vi "Edit Config.vi"(8 "error in (no error)":errorcluster, 11 "Multi Parser in":refnum<class "Mulit Sentence Parser.lvclass">) -> (0 "error out":errorcluster, 3 "Multi Parser out":refnum<class "Mulit Sentence Parser.lvclass">)   [LabVIEW 2018, in "Mulit Sentence Parser.lvclass"]
doc: "Multi Sentence Parser.lvclass:Edit Config.vi\n\nThis VI is used to edit the Multi Sentence Parser configuration parameters.\n\nInstrument Communication Module Version 1.0\nOctober, 2017 Original Code Consulting David Thomson\n www.originalcode.com"
uses:
  Mulit Sentence Parser.lvclass
  Multi Sentence Parser Config.ctl
  Controls/ICM Class Editor State.ctl
  Controls/ICM Editor Command.ctl
  Mulit Sentence Parser.lvclass/Mulit Sentence Parser.ctl
panel:
  in  "Save":bool
  in  "Revert":bool
  in  "Multi Sentence Parser Config":T1
  # "This Parser is intended to be used with devices which send multiple data sentences, potentially at different intervals."
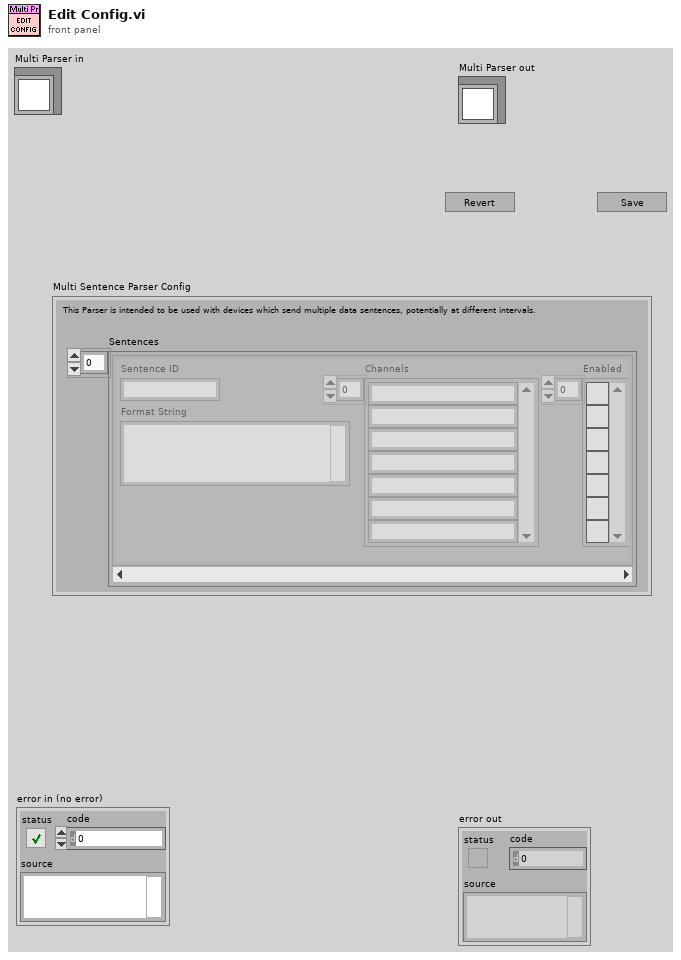
[diagram p1: front panel]
types:
  T1 = typedef "Mulit Sentence Parser.lvclass/Multi Sentence Parser Config.ctl" = cluster{"Sentences":cluster{"Sentence ID":string, "Format String":string, "Channels":string[], "Enabled":bool[]}[]}
  T2 = typedef "ICM Editor Command.ctl" = enum16{"No-op", "Exit"}
  T3 = typedef "ICM Class Editor State.ctl" = enum16{"Init", "Wait", "Write", "Read", "Display", "Set Flashing", "Error", "Stop"}
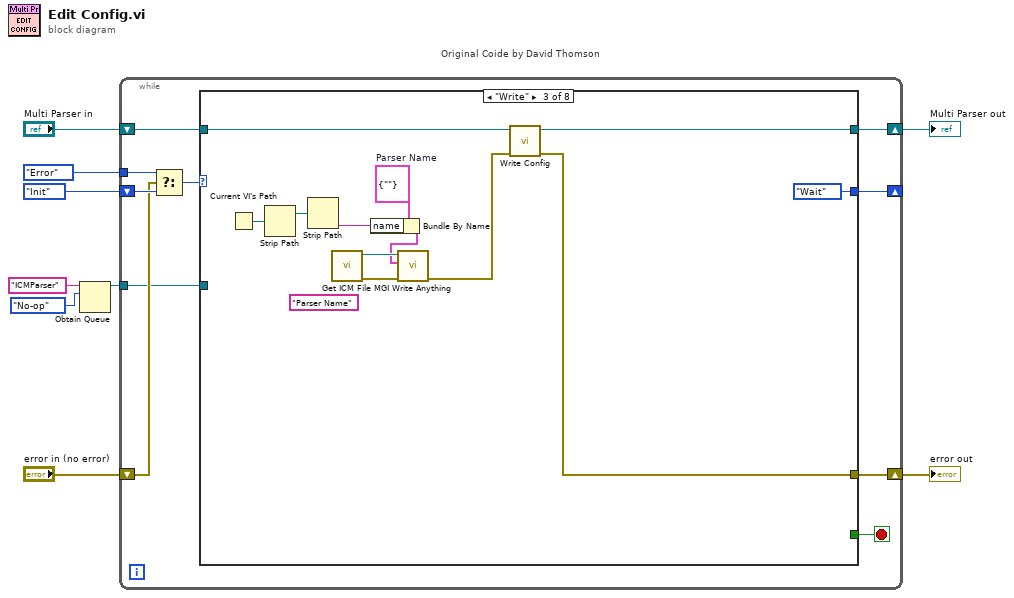
[diagram p0: block diagram]
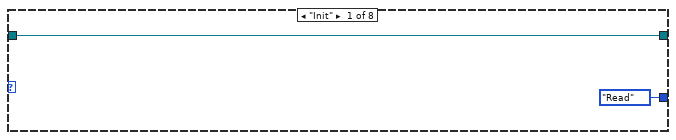
[diagram p2: hidden frame]
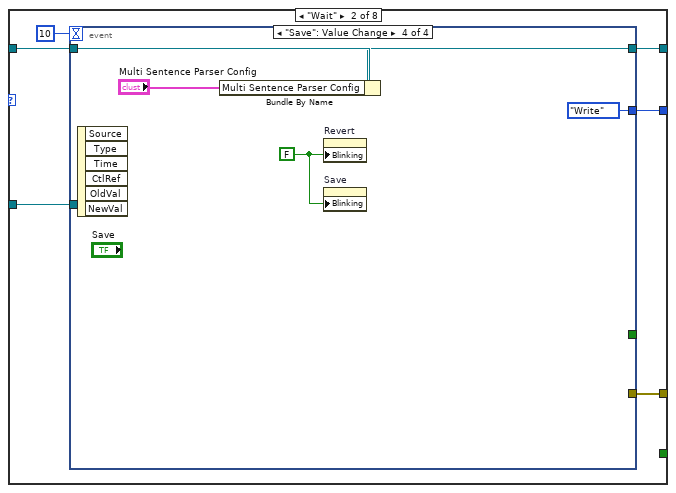
[diagram p3: hidden frame]
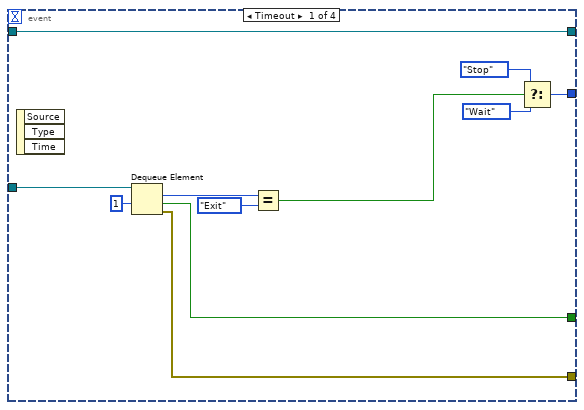
[diagram p4: hidden frame]
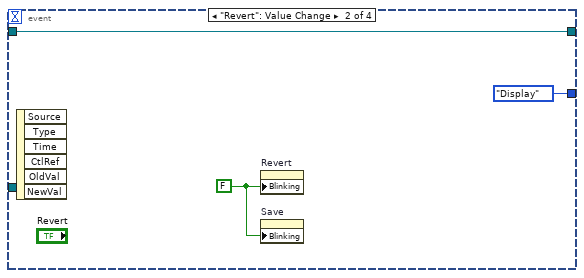
[diagram p5: hidden frame]
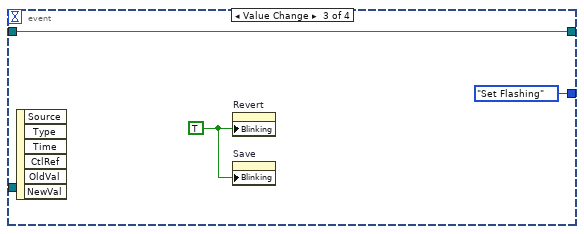
[diagram p6: hidden frame]
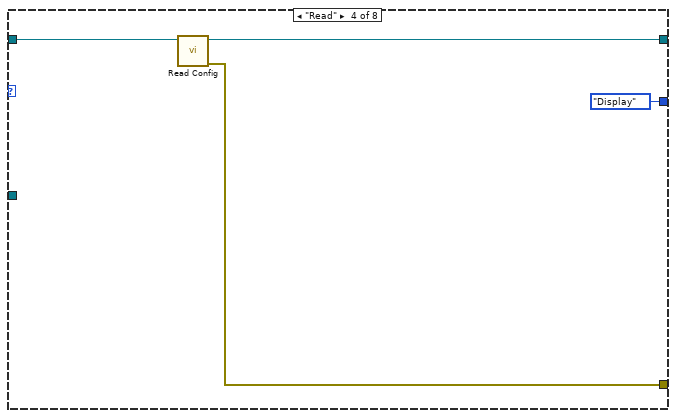
[diagram p7: hidden frame]
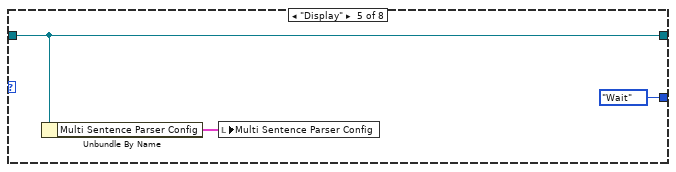
[diagram p8: hidden frame]
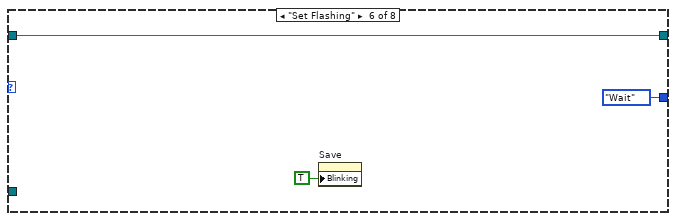
[diagram p9: hidden frame]
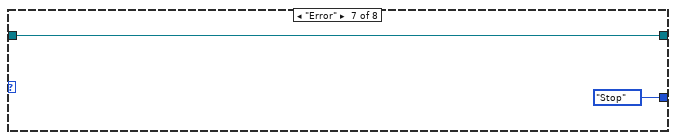
[diagram p10: hidden frame]
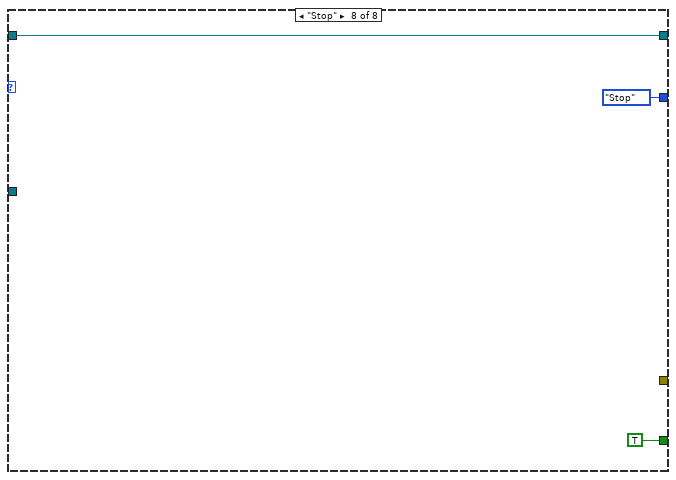
[diagram p11: hidden frame]
diagram:
  n1 = Obtain Queue(name (unnamed)="ICMParser", element data type=ICM_Editor_Command."No-op" ("Editor Command")) -> (queue out=w1:refnum<queue>)  [unwired: 3 in, 2 out]
  n2 = while "Original Coide by David Thomson" {
    shift-right: [w19] -> w8
    shift-left: "Multi Parser in" -> [w18]
    shift-right: [w12] -> _
    shift-left: ICM_Class_Editor_State."Init" ("Config State") -> [w16]
    shift-right: [w11] -> w6
    shift-left: "error in (no error)" -> [w14]
    tunnel: ICM_Class_Editor_State."Error" ("Config State") -> [w13]
    tunnel: w1 -> [w10]
    stop <- w17 stop-if-true
    n3 = Select(t=w13, s=w14, f=w16) -> (s? t:f=w15:T3)
    n4 = case shown="\"Write\"" w15 {
      tunnel: [w20 w25 w59 w63 w68 w71 w73 w76] -> w19
      tunnel: w18 -> [w20 w24 w60 w65 w68 w71 w73 w76]
      tunnel: [_ _ _ _ _ _ _ TRUE] -> w17
      tunnel: [ICM_Class_Editor_State."Read" ("Config State") w26 ICM_Class_Editor_State."Wait" ("Config State") ICM_Class_Editor_State."Display" ("Config State") ICM_Class_Editor_State."Wait" ("Config State") ICM_Class_Editor_State."Wait" ("Config State") ICM_Class_Editor_State."Stop" ("Config State") ICM_Class_Editor_State."Stop" ("Config State")] -> w12
      tunnel: [_ w22 w58 w64 _ _ _ _] -> w11
      tunnel: w10 -> [_ w23 _ _ _ _ _ _]
      frame "Init" {
      }
      frame "Wait" {
        n5 = event shown="[3] \"Save\": Value Change" {
          selector: _ -> [_ _ _ _]
          dyn-events: _ -> [_ _ _ _]
          timeout: 10 -> [_ _ _ _]
          tunnel: [w35 ICM_Class_Editor_State."Display" ("Config State") ICM_Class_Editor_State."Set Flashing" ("Config State") ICM_Class_Editor_State."Write" ("Config State")] -> w26
          tunnel: [w38 w40 w44 w46] -> w25
          tunnel: w24 -> [w38 w40 w44 w47]
          tunnel: w23 -> [w37 _ _ _]
          tunnel: [w29 _ _ _] -> w22
          tunnel: [w28 _ _ _] -> _
          event Timeout {
            n6 = event-data() -> ()  [unwired: 1 in, 3 out]
            n7 = Dequeue Element(queue=w37, timeout in ms (-1)=1) -> (element=w34:T2, timed out?=w28:bool, error out=w29:errorcluster)  [unwired: 1 in, 1 out]
            n8 = Equal?(x=w34, y=ICM_Editor_Command."Exit") -> (x = y?=w32:bool)
            n9 = Select(t=ICM_Class_Editor_State."Stop" ("Config State"), s=w32, f=ICM_Class_Editor_State."Wait" ("Config State")) -> (s? t:f=w35:T3)
          }
          event "Revert": Value Change {
            w39 = FALSE ("Blinking")
            n10 = event-data() -> ()  [unwired: 1 in, 6 out]
            n11 = property on="Revert" class="Bool"("Blinking"=w39) -> ()  [unwired: 2 in, 2 out]
            n12 = property on="Save" class="Bool"("Blinking"=w39) -> ()  [unwired: 2 in, 2 out]
          }
          event Value Change {
            w42 = TRUE ("Blinking")
            n13 = event-data() -> ()  [unwired: 1 in, 6 out]
            n14 = property on="Revert" class="Bool"("Blinking"=w42) -> ()  [unwired: 2 in, 2 out]
            n15 = property on="Save" class="Bool"("Blinking"=w42) -> ()  [unwired: 2 in, 2 out]
          }
          event "Save": Value Change {
            w45 = FALSE ("Blinking")
            n16 = event-data() -> ()  [unwired: 1 in, 6 out]
            n17 = Bundle By Name(cluster=w47, "Multi Sentence Parser Config"="Multi Sentence Parser Config") -> (w46:refnum<class "Mulit Sentence Parser.lvclass">)
            n18 = property on="Revert" class="Bool"("Blinking"=w45) -> ()  [unwired: 2 in, 2 out]
            n19 = property on="Save" class="Bool"("Blinking"=w45) -> ()  [unwired: 2 in, 2 out]
          }
        }
      }
      frame "Write" {
        w52 = cluster{"name":string} {"name"=""}  # Parser Name
        (unwired) "Parser Name" ("Section Name (Name of \"Anything\")")
        n20 = Current VI's Path() -> (path=w57:path)
        n21 = Strip Path(path=w57) -> (stripped path=w56:path)  [unwired: 1 out]
        n22 = Strip Path(path=w56) -> (name=w51:string)  [unwired: 1 out]
        n23 = call "Get ICM File.vi"() -> ("error out"=w54:errorcluster, "ICM File"=w55:path)  [unwired: 10 in]
        n24 = Bundle By Name(cluster=w52, "name"=w51) -> (w50:cluster{"name":string})
        n25 = call <userlib>:"MGI Write Anything.vi"("Error In"=w54, "Anything"=w50, "Path (dialog)"=w55) -> ("Error Out"=w53:errorcluster)  [unwired: 6 in, 2 out]
        n26 = call-dynamic "Write Config.vi"("error in (no error)"=w53, "Multi Parser in"=w60) -> ("error out"=w58:errorcluster, "Multi Parser out"=w59:refnum<class "Mulit Sentence Parser.lvclass">)  [unwired: 8 in]
      }
      frame "Read" {
        n27 = call-dynamic "Read Config.vi"("Multi Parser in"=w65) -> ("error out"=w64:errorcluster, "Multi Parser out"=w63:refnum<class "Mulit Sentence Parser.lvclass">)  [unwired: 9 in]
      }
      frame "Display" {
        n28 = Unbundle By Name(w68) -> ("Multi Sentence Parser Config"=w67:T1)
        n29 = local write "Multi Sentence Parser Config"(w67) -> ()
      }
      frame "Set Flashing" {
        n30 = property on="Save" class="Bool"("Blinking"=TRUE) -> ()  [unwired: 2 in, 2 out]
      }
      frame "Error" {
      }
      frame "Stop" {
      }
    }
  }
  "error out" <- w6
  "Multi Parser out" <- w8
